vi "Main.vi"() -> ()   [LabVIEW 2019]
doc: "This template is for the Queued Message Handler design pattern.\n\nThe Event Handling Loop generates messages based on user interface actions.\n\nThe Message Handling Loop processes messages generated by the Event Handling Loop, or by other messages. The messages are string values, so new messages can be added easily to the Message Cases case structure in the Message Handling Loop. Each message cluster can also provide an optional value for Message Data, which is a variant that can be converted to whatever message-specific data is required."
uses:
  controls/UI Data.ctl
  support/Message Queue/Message Queue.lvlib
  <vilib>/Utility/error.llb/Error Cluster From Error Code.vi
  support/User Event - Stop/User Event - Stop.lvlib
  support/Message Queue/Enqueue Message (Single).vi
  <vilib>/ErrorRing/Error Ring.xnode
  <vilib>/Analysis/NI_AALBase.lvlib
  <vilib>/Instr/_visa.llb/VISA Configure Serial Port (Instr).vi
panel:
  in  "?":enum32{"PLSC-21/LDP-V", "BFS-VRM 03"}(tab)
  in  "Set Max. Duty Cycle":dbl
  out "Duty Cycle":dbl(slide) scale=0.0..0.15
  in  "Exit":bool
  in  "Start Laser":bool
  in  "Stop Laser":bool
  out "Display (Code)":string
  in  "Pulse Length (ns)":dbl(slide) scale=8.0..100.0
  in  "Set Pulse Length":bool
  in  "Voltage (mv)":dbl(slide) scale=0.0..10000.0
  in  "Set Precharger Voltage":bool
  in  "Rep. Rate (Hz)":dbl(slide) scale=0.0..1000.0
  in  "Modes":enum32{"Voltage Mode", "Current Mode"}(radio)
  in  "Current":u64(knob) scale=0.0..100.0
  out "Waveform":dbl[](graph)
  in  "Sample Rate":i32(slide) scale=0.0..8000.0
  out "LED":bool=TRUE
  in  "Save Settings\nPLCS":bool
  in  "Load Settings\nPLCS":bool
  in  "Save Settings BFS":bool
  in  "TEC Current Limit (A)":dbl(slide) scale=0.0..1.0
  in  "TEC KI":dbl(slide) scale=0.0..0.04
  in  "TEC KP":dbl(slide) scale=0.0..2.0
  in  "TEC Temperatur":dbl(knob) scale=0.0..70.0
  in  "VREF (V)":dbl(slide) scale=0.0..1.0
  in  "Load Settings BFS":bool
  out "Display (Code)":string
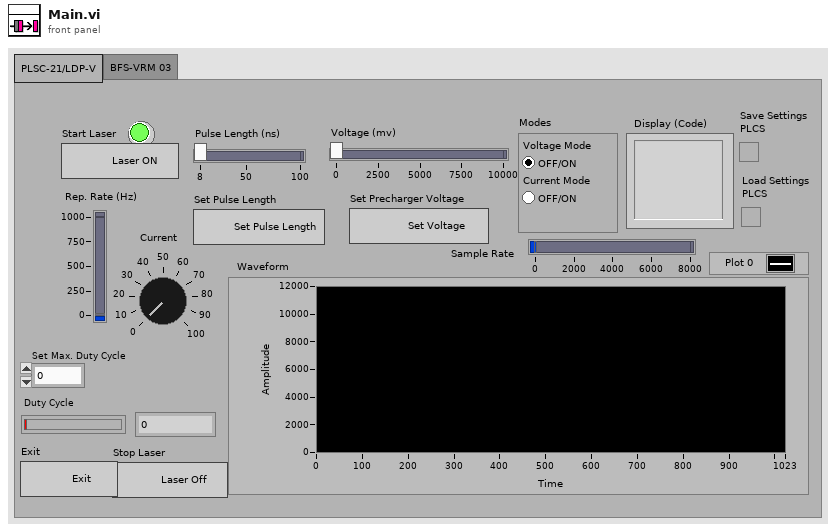
[diagram p1: front panel]
types:
  T1 = typedef "UI Data.ctl" = cluster{"Boolean <Replace Me>":bool, "String <Replace Me>":string, "Numeric <Replace Me>":dbl, "Do Something Ref":refnum<vi>, "Do Something Else Ref":refnum<vi>, "Data Display Ref":refnum<vi>, "Exit Button Ref":refnum<vi>}
  T2 = typedef "Message Queue.lvlib/All Message Queues.ctl" = cluster{"UI":refnum<queue>}
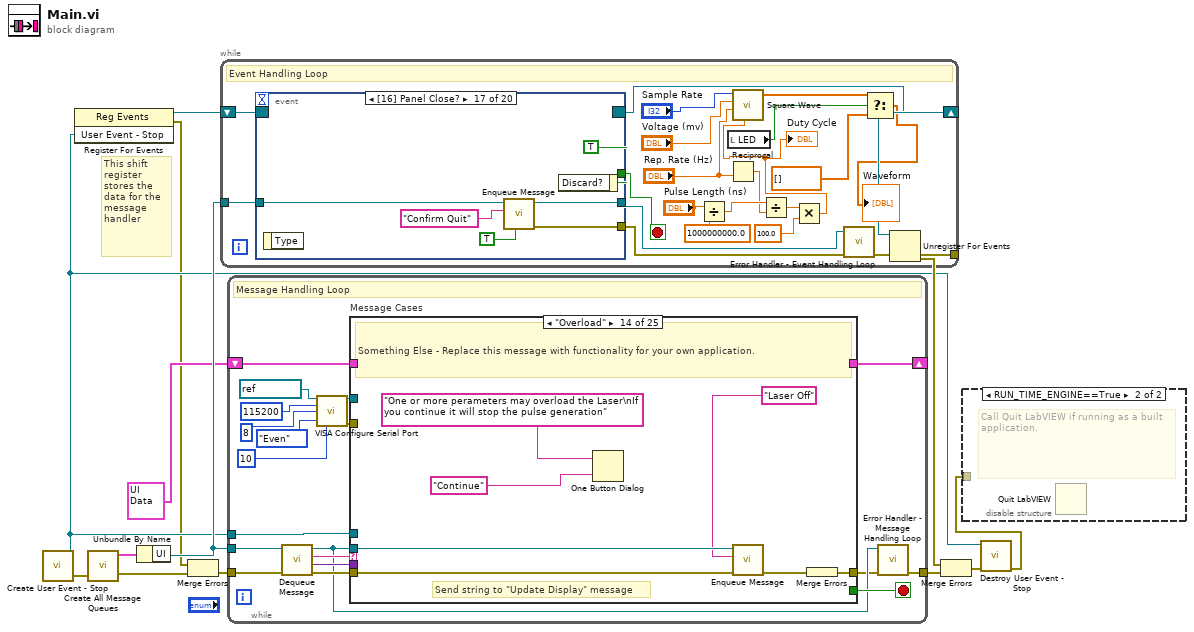
[diagram p0: block diagram]
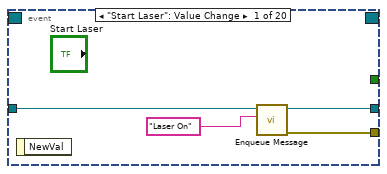
[diagram p3: hidden frame]
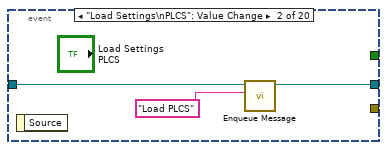
[diagram p4: hidden frame]
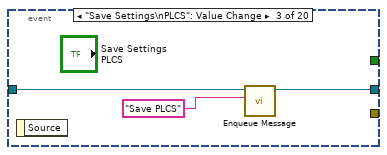
[diagram p5: hidden frame]
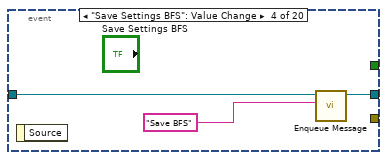
[diagram p6: hidden frame]
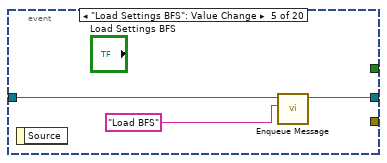
[diagram p7: hidden frame]
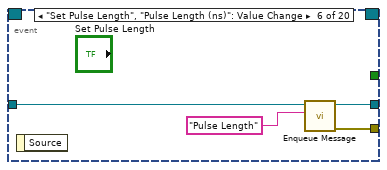
[diagram p8: hidden frame]
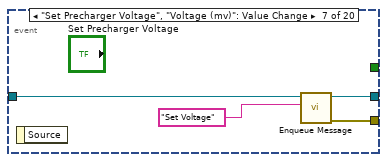
[diagram p9: hidden frame]
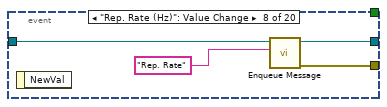
[diagram p10: hidden frame]
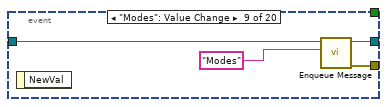
[diagram p11: hidden frame]
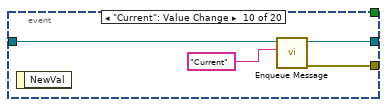
[diagram p12: hidden frame]
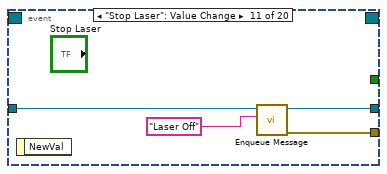
[diagram p13: hidden frame]
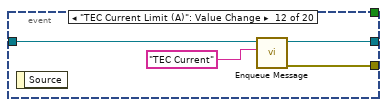
[diagram p14: hidden frame]
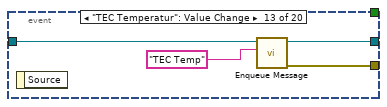
[diagram p15: hidden frame]
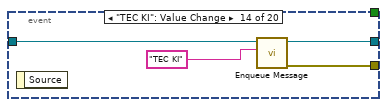
[diagram p16: hidden frame]
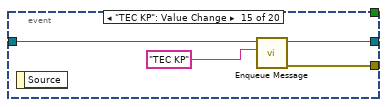
[diagram p17: hidden frame]
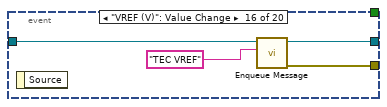
[diagram p18: hidden frame]
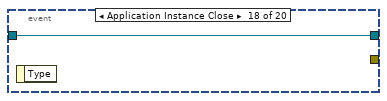
[diagram p19: hidden frame]
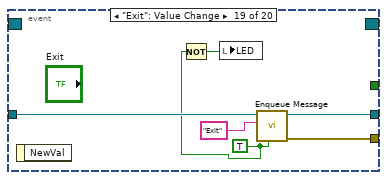
[diagram p20: hidden frame]
diagram:
  # "This shift register stores the data for the message handler"
  n1 = call "Create User Event - Stop.vi"() -> ("error out"=w11:errorcluster, "User Event - Stop"=w4:refnum<user-event>)  [unwired: 10 in]
  n2 = register-events(w4) -> (reference out=w5:refnum<event-registration>, error out=w2:errorcluster)  [unwired: 2 in]
  n3 = call "Create All Message Queues.vi"("error in (no error)"=w11) -> ("error out"=w15:errorcluster, "Message Queues out"=w14:T2)  [unwired: 9 in]
  n4 = Unbundle By Name(w14) -> ("UI"=w12:refnum<queue>)
  n5 = Merge Errors(w2, w15) -> (w3:errorcluster)
  n6 = while {
    tunnel: w12 -> [w36]
    shift-right: [w31] -> w8
    shift-left: w5 -> [w35]
    tunnel: [w33] -> w6
    stop <- w30 stop-if-true
    # "Event Handling Loop"
    n7 = event shown="[16] Panel Close?" {
      selector: w35 -> [_ _ _ _ _ _ _ _ _ _ _ _ _ _ _ _ _ _ _ _]
      dyn-events: [_ _ _ _ _ _ _ _ _ _ _ _ _ _ _ _ _ _ _ _] -> w31
      timeout: _ -> [_ _ _ _ _ _ _ _ _ _ _ _ _ _ _ _ _ _ _ _]
      tunnel: [_ _ _ _ _ _ _ _ _ _ _ _ _ _ _ _ _ _ _ TRUE ("Discard?")] -> w30
      tunnel: w36 -> [w40 w43 w46 w48 w51 w55 w60 w64 w68 w72 w76 w80 w84 w88 w92 w96 w101 w103 w109 w112]
      tunnel: [w37 _ _ _ _ w53 w58 w61 w65 w70 w73 w77 w81 w85 w89 w93 w100 _ w108 _] -> w34
      tunnel: [w39 w42 w45 w49 w52 w54 w59 w63 w67 w71 w75 w79 w83 w87 w91 w95 w99 w103 w107 w112] -> w32
      event "Start Laser": Value Change {
        n8 = event-data() -> ()  [unwired: 1 in, 1 out]
        n9 = call-poly "Enqueue Message.vi"("Message"="Laser On", "Message Queue"=w40) -> ("error out"=w37:errorcluster, "dup Message Queue"=w39:refnum<queue>)  [unwired: 8 in]
      }
      event "Load Settings\nPLCS": Value Change {
        n10 = event-data() -> ()  [unwired: 1 in, 1 out]
        n11 = call-poly "Enqueue Message.vi"("Message"="Load PLCS", "Message Queue"=w43) -> ("dup Message Queue"=w42:refnum<queue>)  [unwired: 8 in, 1 out]
      }
      event "Save Settings\nPLCS": Value Change {
        n12 = event-data() -> ()  [unwired: 1 in, 1 out]
        n13 = call-poly "Enqueue Message.vi"("Message"="Save PLCS", "Message Queue"=w46) -> ("dup Message Queue"=w45:refnum<queue>)  [unwired: 8 in, 1 out]
      }
      event "Save Settings BFS": Value Change {
        n14 = event-data() -> ()  [unwired: 1 in, 1 out]
        n15 = call-poly "Enqueue Message.vi"("Message"="Save BFS", "Message Queue"=w48) -> ("dup Message Queue"=w49:refnum<queue>)  [unwired: 8 in, 1 out]
      }
      event "Load Settings BFS": Value Change {
        n16 = event-data() -> ()  [unwired: 1 in, 1 out]
        n17 = call-poly "Enqueue Message.vi"("Message"="Load BFS", "Message Queue"=w51) -> ("dup Message Queue"=w52:refnum<queue>)  [unwired: 8 in, 1 out]
      }
      event "Set Pulse Length", "Pulse Length (ns)": Value Change {
        n18 = event-data() -> ()  [unwired: 1 in, 1 out]
        n19 = call-poly "Enqueue Message.vi"("Message"="Pulse Length", "Message Queue"=w55) -> ("error out"=w53:errorcluster, "dup Message Queue"=w54:refnum<queue>)  [unwired: 8 in]
      }
      event "Set Precharger Voltage", "Voltage (mv)": Value Change {
        n20 = event-data() -> ()  [unwired: 1 in, 1 out]
        n21 = call-poly "Enqueue Message.vi"("Message"="Set Voltage", "Message Queue"=w60) -> ("error out"=w58:errorcluster, "dup Message Queue"=w59:refnum<queue>)  [unwired: 8 in]
      }
      event "Rep. Rate (Hz)": Value Change {
        n22 = event-data() -> ()  [unwired: 1 in, 1 out]
        n23 = call-poly "Enqueue Message.vi"("Message"="Rep. Rate", "Message Queue"=w64) -> ("error out"=w61:errorcluster, "dup Message Queue"=w63:refnum<queue>)  [unwired: 8 in]
      }
      event "Modes": Value Change {
        n24 = event-data() -> ()  [unwired: 1 in, 1 out]
        n25 = call-poly "Enqueue Message.vi"("Message"="Modes", "Message Queue"=w68) -> ("error out"=w65:errorcluster, "dup Message Queue"=w67:refnum<queue>)  [unwired: 8 in]
      }
      event "Current": Value Change {
        n26 = event-data() -> ()  [unwired: 1 in, 1 out]
        n27 = call-poly "Enqueue Message.vi"("Message"="Current", "Message Queue"=w72) -> ("error out"=w70:errorcluster, "dup Message Queue"=w71:refnum<queue>)  [unwired: 8 in]
      }
      event "Stop Laser": Value Change {
        n28 = event-data() -> ()  [unwired: 1 in, 1 out]
        n29 = call-poly "Enqueue Message.vi"("Message"="Laser Off", "Message Queue"=w76) -> ("error out"=w73:errorcluster, "dup Message Queue"=w75:refnum<queue>)  [unwired: 8 in]
      }
      event "TEC Current Limit (A)": Value Change {
        n30 = event-data() -> ()  [unwired: 1 in, 1 out]
        n31 = call-poly "Enqueue Message.vi"("Message"="TEC Current", "Message Queue"=w80) -> ("error out"=w77:errorcluster, "dup Message Queue"=w79:refnum<queue>)  [unwired: 8 in]
      }
      event "TEC Temperatur": Value Change {
        n32 = event-data() -> ()  [unwired: 1 in, 1 out]
        n33 = call-poly "Enqueue Message.vi"("Message"="TEC Temp", "Message Queue"=w84) -> ("error out"=w81:errorcluster, "dup Message Queue"=w83:refnum<queue>)  [unwired: 8 in]
      }
      event "TEC KI": Value Change {
        n34 = event-data() -> ()  [unwired: 1 in, 1 out]
        n35 = call-poly "Enqueue Message.vi"("Message"="TEC KI", "Message Queue"=w88) -> ("error out"=w85:errorcluster, "dup Message Queue"=w87:refnum<queue>)  [unwired: 8 in]
      }
      event "TEC KP": Value Change {
        n36 = event-data() -> ()  [unwired: 1 in, 1 out]
        n37 = call-poly "Enqueue Message.vi"("Message"="TEC KP", "Message Queue"=w92) -> ("error out"=w89:errorcluster, "dup Message Queue"=w91:refnum<queue>)  [unwired: 8 in]
      }
      event "VREF (V)": Value Change {
        n38 = event-data() -> ()  [unwired: 1 in, 1 out]
        n39 = call-poly "Enqueue Message.vi"("Message"="TEC VREF", "Message Queue"=w96) -> ("error out"=w93:errorcluster, "dup Message Queue"=w95:refnum<queue>)  [unwired: 8 in]
      }
      event Panel Close? {
        n40 = event-data() -> ()  [unwired: 1 in, 1 out]
        n41 = call-poly "Enqueue Message.vi"("Priority Message? (F)"=TRUE, "Message"="Confirm Quit", "Message Queue"=w101) -> ("error out"=w100:errorcluster, "dup Message Queue"=w99:refnum<queue>)  [unwired: 7 in]
        n42 = event-data("Discard?"=TRUE) -> ()  [unwired: 1 in, 1 out]
      }
      event Application Instance Close {
        n43 = event-data() -> ()  [unwired: 1 in, 1 out]
      }
      event "Exit": Value Change {
        w104 = TRUE ("Priority Message? (F)")
        n44 = event-data() -> ()  [unwired: 1 in, 1 out]
        n45 = Not(x=w104) -> (.not. x?=w105:bool)
        n46 = local write "LED"(w105) -> ()
        n47 = call-poly "Enqueue Message.vi"("Priority Message? (F)"=w104, "Message"="Exit", "Message Queue"=w109) -> ("error out"=w108:errorcluster, "dup Message Queue"=w107:refnum<queue>)  [unwired: 7 in]
      }
      event User Event {
        n48 = event-data() -> ()  [unwired: 1 in, 1 out]
        n49 = local write "Display (Code)"("\"Exit\" button pressed/COM Released" ("VI Stopped")) -> ()
      }
    }
    n50 = Divide(x="Pulse Length (ns)", y=1000000000.0) -> (x/y=w26:dbl)
    n51 = local read "LED"() -> (w19:bool)
    n52 = Reciprocal(x="Rep. Rate (Hz)") -> (1/x=w25:dbl)
    n53 = Divide(x=w26, y=w25) -> (x/y=w24:dbl)
    n54 = Multiply(x=w24, y=100.0) -> (x*y=w17:dbl)
    "Duty Cycle" <- w17
    n55 = call <vilib>:"Square Wave.vi"("samples"="Sample Rate", "amplitude"="Voltage (mv)", "frequency"="Rep. Rate (Hz)", "duty cycle (%)"=w17) -> ("square wave"=w20:dbl[])  [unwired: 2 in, 2 out]
    n56 = call "Error Handler - Event Handling Loop.vi"("error in (no error)"=w34, "Message Queue"=w32) -> ("dup error in"=w33:errorcluster)  [unwired: 8 in, 1 out]
    n57 = Select(t=w20, s=w19, f=dbl[] [] ("History Data")) -> (s? t:f=→"Waveform":dbl[])
  }
  n58 = while {
    tunnel: w12 -> [w123]
    shift-right: [w130] -> _
    shift-left: T1 {"Boolean <Replace Me>"=FALSE, "String <Replace Me>"="", "Numeric <Replace Me>"=0.0, "Do Something Ref"=refnum, "Do Something Else Ref"=refnum, "Data Display Ref"=refnum, "Exit Button Ref"=refnum} ("Data Cluster") -> [w131]
    tunnel: w4 -> [w128]
    tunnel: w3 -> [w127]
    tunnel: [w121] -> w13
    stop <- w129 stop-if-true
    # "Message Handling Loop"
    n59 = call "Dequeue Message.vi"("error in (no error)"=w127, "Message Queue"=w123) -> ("error out"=w126:errorcluster, "Message Data"=w124:variant, "Message"=w125:string, "dup Message Queue"=w122:refnum<queue>)  [unwired: 6 in]
    n60 = call-poly "VISA Configure Serial Port"("VISA resource name"=refnum<visa-resource-name> "COM4", "baud rate (9600)"=u32 115200, "data bits (8)"=u16 8, "parity (0:none)"=enum16{"None", "Odd", "Even", "Mark", "Space"}."Even", "stop bits (10: 1 bit)"=u16 10) -> ("VISA resource name out"=w114:refnum<visa-resource-name>, "error out"=w113:errorcluster)  [unwired: 9 in]
    n61 = case "Message Cases" shown="\"Overload\"" w125 {
      selector: w125 -> [_ _ _ _ _ _ _ _ _ _ _ _ _ _ _ _ _ _ _ _ _ _ _ _ w434]
      tunnel: w122 -> [w136 w160 w175 w195 w214 w220 w245 w263 w281 w299 w317 w330 w344 w352 _ _ _ _ _ _ _ w412 _ w433 _]
      tunnel: w126 -> [w144 w161 w177 w197 w216 w222 w247 w265 w283 w301 w319 w332 w346 w354 w364 w372 w380 w388 w393 w400 w409 w416 w419 w426 _]
      tunnel: [w145 w163 w176 w196 w215 w221 w246 w264 w282 w300 w318 w333 w347 w355 w364 w372 w380 w388 w394 w401 w403 w414 w417 w429 w435] -> w120
      tunnel: w131 -> [w143 w147 w180 w185 w219 w231 w249 w267 w285 w303 w321 w334 w348 w356 w363 w371 w379 w387 w395 w402 w408 w415 w418 w432 w436]
      tunnel: [w142 w147 w180 w185 w219 w231 w249 w267 w285 w303 w321 w334 w348 w356 w363 w371 w379 w387 w395 w402 w408 w415 w418 w432 w436] -> w130
      tunnel: [_ _ _ _ _ _ _ _ _ _ _ _ _ _ _ _ _ _ _ _ _ _ _ TRUE _] -> w129
      tunnel: w124 -> [_ _ _ _ _ _ _ _ _ _ _ _ _ _ _ _ _ _ w392 w399 w407 _ _ w423 _]
      tunnel: w128 -> [_ _ _ _ _ _ _ _ _ _ _ _ _ _ _ _ _ _ _ _ _ _ _ w428 _]
      tunnel: w114 -> [_ w168 w179 w203 w213 w230 _ _ _ _ _ w328 w340 _ _ _ _ _ _ _ _ _ _ w422 _]
      tunnel: w113 -> [_ w167 w178 w202 w212 w229 _ _ _ _ _ w327 w339 _ _ _ _ _ _ _ _ _ _ w421 _]
      frame "Initialize" {
        w132 = "Initial Message" ("Initial Message")
        # "Bundle control references and a sample string value."
        # "Initialize - All initialization work should take place in this message, since other loops can potentially enqueue messages that execute immediately after this one."
        n62 = control-ref of="Start Laser"() -> (w141:refnum<vi>)
        n63 = control-ref of="Stop Laser"() -> (w140:refnum<vi>)
        n64 = control-ref of="Exit"() -> (w138:refnum<vi>)
        n65 = control-ref of="Display (Code)"() -> (w139:refnum<vi>)
        n66 = String Length(string=w132) -> (length=w134:i32)
        n67 = Less Than 0?(x=w134) -> (x < 0?=w133:bool)
        n68 = Bundle By Name(cluster=w143, "Do Something Ref"=w141, "Do Something Else Ref"=w140, "Data Display Ref"=w139, "Exit Button Ref"=w138, "String <Replace Me>"=w132) -> (w142:T1)
        n69 = local write "LED"(w133) -> ()
        n70 = property on="Waveform" class="WFChart (strict)"("History Data"=dbl[] []) -> ()  [unwired: 2 in, 2 out]
        n71 = call-poly "Enqueue Message.vi"("error in (no error)"=w144, "Message Data"=w132, "Message"="Update Display", "Message Queue"=w136) -> ("error out"=w145:errorcluster)  [unwired: 6 in, 1 out]
      }
      frame "Pulse Length" {
        n72 = local read "Pulse Length (ns)"() -> (w162:dbl)
        n73 = local read "Duty Cycle"() -> (w154:dbl)
        n74 = Concatenate Strings("Laseroff" ("Message"), "\r") -> (w148:string)
        n75 = Number To Decimal String(number=w162) -> (decimal integer string=w165:string)  [unwired: 1 in]
        n76 = Greater Or Equal?(x=w154, y="Set Max. Duty Cycle") -> (x >= y?=w155:bool)
        n77 = In Range and Coerce(upper limit="Set Max. Duty Cycle", x=w154, lower limit=0.0) -> (In Range?=w158:bool)  [unwired: 1 out]
        n78 = Select(t="Overload" ("Message"), s=w155, f="Update Display" ("Message")) -> (s? t:f=w153:string)
        n79 = Concatenate Strings("spulse ", w165, "\r") -> (w157:string)
        n80 = Select(t=w157, s=w158, f=w148) -> (s? t:f=w156:string)
        n81 = VISA Write(VISA resource name=w168, write buffer=w156, error in (no error)=w167) -> ()  [unwired: 3 out]
        n82 = call-poly "Enqueue Message.vi"("error in (no error)"=w161, "Message Data"=w156, "Message"=w153, "Message Queue"=w160) -> ("error out"=w163:errorcluster)  [unwired: 6 in, 1 out]
      }
      frame "Set Voltage" {
        n83 = local read "Voltage (mv)"() -> (w169:dbl)
        n84 = Number To Decimal String(number=w169) -> (decimal integer string=w172:string)  [unwired: 1 in]
        n85 = Concatenate Strings("svoltage  ", w172, "\r") -> (w170:string)
        n86 = VISA Write(VISA resource name=w179, write buffer=w170, error in (no error)=w178) -> ()  [unwired: 3 out]
        n87 = call-poly "Enqueue Message.vi"("error in (no error)"=w177, "Message Data"=w170, "Message"="Update Display", "Message Queue"=w175) -> ("error out"=w176:errorcluster)  [unwired: 6 in, 1 out]
      }
      frame "Rep. Rate" {
        n88 = local read "Set Max. Duty Cycle"() -> (w181:dbl)
        n89 = local read "Rep. Rate (Hz)"() -> (w198:dbl)
        n90 = local read "Duty Cycle"() -> (w186:dbl)
        n91 = In Range and Coerce(upper limit=w181, x=w186, lower limit=0.0) -> (In Range?=w193:bool)  [unwired: 1 out]
        n92 = Concatenate Strings("laseroff ", "\r") -> (w189:string)
        n93 = Number To Decimal String(number=w198) -> (decimal integer string=w200:string)  [unwired: 1 in]
        n94 = Greater Or Equal?(x=w186, y=w181) -> (x >= y?=w187:bool)
        n95 = Select(t="Overload" ("Message"), s=w187, f="Update Display" ("Message")) -> (s? t:f=w183:string)
        n96 = Concatenate Strings("sreprate  ", w200, "\r") -> (w192:string)
        n97 = Select(t=w192, s=w193, f=w189) -> (s? t:f=w188:string)
        n98 = VISA Write(VISA resource name=w203, write buffer=w188, error in (no error)=w202) -> ()  [unwired: 3 out]
        n99 = call-poly "Enqueue Message.vi"("error in (no error)"=w197, "Message Data"=w188, "Message"=w183, "Message Queue"=w195) -> ("error out"=w196:errorcluster)  [unwired: 6 in, 1 out]
      }
      frame "Modes" {
        n100 = Equal To 0?(x="Modes") -> (x = 0?=w218:bool)
        n101 = Select(t=1, s=w218, f=2) -> (s? t:f=w209:i32)
        n102 = Number To Decimal String(number=w209) -> (decimal integer string=w208:string)  [unwired: 1 in]
        n103 = Concatenate Strings("smode ", w208, "\r") -> (w204:string)
        n104 = VISA Write(VISA resource name=w213, write buffer=w204, error in (no error)=w212) -> ()  [unwired: 3 out]
        n105 = call-poly "Enqueue Message.vi"("error in (no error)"=w216, "Message Data"=w204, "Message"="Update Display", "Message Queue"=w214) -> ("error out"=w215:errorcluster)  [unwired: 6 in, 1 out]
      }
      frame "Current" {
        n106 = Number To Decimal String(number="Current") -> (decimal integer string=w228:string)  [unwired: 1 in]
        n107 = Concatenate Strings("scurrent  ", w228, "\r") -> (w224:string)
        n108 = VISA Write(VISA resource name=w230, write buffer=w224, error in (no error)=w229) -> ()  [unwired: 3 out]
        n109 = call-poly "Enqueue Message.vi"("error in (no error)"=w222, "Message Data"=w224, "Message"="Update Display", "Message Queue"=w220) -> ("error out"=w221:errorcluster)  [unwired: 6 in, 1 out]
      }
      frame "TEC Current" {
        n110 = local read "TEC Current Limit (A)"() -> (w244:dbl)
        n111 = call-poly "VISA Configure Serial Port"("VISA resource name"=refnum<visa-resource-name> "COM3", "baud rate (9600)"=u32 115200, "data bits (8)"=u16 8, "parity (0:none)"=enum16{"None", "Odd", "Even", "Mark", "Space"}."Even", "stop bits (10: 1 bit)"=u16 10) -> ("VISA resource name out"=w233:refnum<visa-resource-name>, "error out"=w232:errorcluster)  [unwired: 9 in]
        n112 = Number To Fractional String(number=w244, precision (6)=2) -> (F-format string=w243:string)  [unwired: 2 in]
        n113 = Concatenate Strings("simax  ", w243, "\r") -> (w239:string)
        n114 = VISA Write(VISA resource name=w233, write buffer=w239, error in (no error)=w232) -> ()  [unwired: 3 out]
        n115 = call-poly "Enqueue Message.vi"("error in (no error)"=w247, "Message Data"=w239, "Message"="Display 2", "Message Queue"=w245) -> ("error out"=w246:errorcluster)  [unwired: 6 in, 1 out]
      }
      frame "TEC Temp" {
        w259 = "stsoll  "  # stsoll
        n116 = local read "TEC Temperatur"() -> (w262:dbl)
        n117 = call-poly "VISA Configure Serial Port"("VISA resource name"=refnum<visa-resource-name> "COM3", "baud rate (9600)"=u32 115200, "data bits (8)"=u16 8, "parity (0:none)"=enum16{"None", "Odd", "Even", "Mark", "Space"}."Even", "stop bits (10: 1 bit)"=u16 10) -> ("VISA resource name out"=w251:refnum<visa-resource-name>, "error out"=w250:errorcluster)  [unwired: 9 in]
        n118 = Number To Fractional String(number=w262, precision (6)=0) -> (F-format string=w261:string)  [unwired: 2 in]
        n119 = Concatenate Strings(w259, w261, "\r") -> (w257:string)
        n120 = VISA Write(VISA resource name=w251, write buffer=w257, error in (no error)=w250) -> ()  [unwired: 3 out]
        n121 = call-poly "Enqueue Message.vi"("error in (no error)"=w265, "Message Data"=w257, "Message"="Display 2", "Message Queue"=w263) -> ("error out"=w264:errorcluster)  [unwired: 6 in, 1 out]
      }
      frame "TEC KI" {
        w277 = "ski  "  # ski
        n122 = local read "TEC KI"() -> (w280:dbl)
        n123 = call-poly "VISA Configure Serial Port"("VISA resource name"=refnum<visa-resource-name> "COM3", "baud rate (9600)"=u32 115200, "data bits (8)"=u16 8, "parity (0:none)"=enum16{"None", "Odd", "Even", "Mark", "Space"}."Even", "stop bits (10: 1 bit)"=u16 10) -> ("VISA resource name out"=w269:refnum<visa-resource-name>, "error out"=w268:errorcluster)  [unwired: 9 in]
        n124 = Number To Fractional String(number=w280, precision (6)=2) -> (F-format string=w279:string)  [unwired: 2 in]
        n125 = Concatenate Strings(w277, w279, "\r") -> (w275:string)
        n126 = VISA Write(VISA resource name=w269, write buffer=w275, error in (no error)=w268) -> ()  [unwired: 3 out]
        n127 = call-poly "Enqueue Message.vi"("error in (no error)"=w283, "Message Data"=w275, "Message"="Display 2", "Message Queue"=w281) -> ("error out"=w282:errorcluster)  [unwired: 6 in, 1 out]
      }
      frame "TEC KP" {
        w295 = "skp  "  # skp
        n128 = local read "TEC KP"() -> (w298:dbl)
        n129 = call-poly "VISA Configure Serial Port"("VISA resource name"=refnum<visa-resource-name> "COM3", "baud rate (9600)"=u32 115200, "data bits (8)"=u16 8, "parity (0:none)"=enum16{"None", "Odd", "Even", "Mark", "Space"}."Even", "stop bits (10: 1 bit)"=u16 10) -> ("VISA resource name out"=w287:refnum<visa-resource-name>, "error out"=w286:errorcluster)  [unwired: 9 in]
        n130 = Number To Fractional String(number=w298, precision (6)=2) -> (F-format string=w297:string)  [unwired: 2 in]
        n131 = Concatenate Strings(w295, w297, "\r") -> (w293:string)
        n132 = VISA Write(VISA resource name=w287, write buffer=w293, error in (no error)=w286) -> ()  [unwired: 3 out]
        n133 = call-poly "Enqueue Message.vi"("error in (no error)"=w301, "Message Data"=w293, "Message"="Display 2", "Message Queue"=w299) -> ("error out"=w300:errorcluster)  [unwired: 6 in, 1 out]
      }
      frame "TEC VREF" {
        w313 = "svref "  # svref
        n134 = local read "VREF (V)"() -> (w316:dbl)
        n135 = call-poly "VISA Configure Serial Port"("VISA resource name"=refnum<visa-resource-name> "COM3", "baud rate (9600)"=u32 115200, "data bits (8)"=u16 8, "parity (0:none)"=enum16{"None", "Odd", "Even", "Mark", "Space"}."Even", "stop bits (10: 1 bit)"=u16 10) -> ("VISA resource name out"=w305:refnum<visa-resource-name>, "error out"=w304:errorcluster)  [unwired: 9 in]
        n136 = Number To Fractional String(number=w316, precision (6)=2) -> (F-format string=w315:string)  [unwired: 2 in]
        n137 = Concatenate Strings(w313, w315, "\r") -> (w311:string)
        n138 = VISA Write(VISA resource name=w305, write buffer=w311, error in (no error)=w304) -> ()  [unwired: 3 out]
        n139 = call-poly "Enqueue Message.vi"("error in (no error)"=w319, "Message Data"=w311, "Message"="Display 2", "Message Queue"=w317) -> ("error out"=w318:errorcluster)  [unwired: 6 in, 1 out]
      }
      frame "Laser On" {
        # "Send string to \"Update Display\" message"
        # "Something - Replace this message with functionality for your own application."
        n140 = Concatenate Strings("laseron", "\r") -> (w323:string)
        n141 = String Length(string=w323) -> (length=w322:i32)
        n142 = VISA Write(VISA resource name=w328, write buffer=w323, error in (no error)=w327) -> ()  [unwired: 3 out]
        n143 = Greater Than 0?(x=w322) -> (x > 0?=→"LED":bool)
        n144 = call-poly "Enqueue Message.vi"("error in (no error)"=w332, "Message Data"=w323, "Message"="Update Display", "Message Queue"=w330) -> ("error out"=w331:errorcluster)  [unwired: 6 in, 1 out]
        n145 = Merge Errors(w331) -> (w333:errorcluster)
      }
      frame "Laser Off" {
        # "Send string to \"Update Display\" message"
        # "Something Else - Replace this message with functionality for your own application."
        n146 = Concatenate Strings("laseroff", "\r") -> (w335:string)
        n147 = VISA Write(VISA resource name=w340, write buffer=w335, error in (no error)=w339) -> ()  [unwired: 3 out]
        n148 = String Length(string=w335) -> (length=w337:i32)
        n149 = Less Than 0?(x=w337) -> (x < 0?=w336:bool)
        n150 = local write "LED"(w336) -> ()
        n151 = call-poly "Enqueue Message.vi"("error in (no error)"=w346, "Message Data"=w335, "Message"="Update Display", "Message Queue"=w344) -> ("error out"=w345:errorcluster)  [unwired: 6 in, 1 out]
        n152 = property on="Waveform" class="WFChart (strict)"("History Data"=dbl[] []) -> ()  [unwired: 2 in, 2 out]
        n153 = Merge Errors(w345) -> (w347:errorcluster)
      }
      frame "Overload" {
        # "Send string to \"Update Display\" message"
        # "Something Else - Replace this message with functionality for your own application."
        n154 = One Button Dialog(message="One or more perameters may overload the Laser\nIf you continue it will stop the pulse generation" ("Message"), button name ("OK")="Continue" ("Message")) -> ()  [unwired: 1 out]
        n155 = call-poly "Enqueue Message.vi"("error in (no error)"=w354, "Message"="Laser Off", "Message Queue"=w352) -> ("error out"=w353:errorcluster)  [unwired: 7 in, 1 out]
        n156 = Merge Errors(w353) -> (w355:errorcluster)
      }
      frame "Save BFS" {
        n157 = Merge Signals("TEC Temperatur", "VREF (V)", "TEC KI", "TEC KP", "TEC Current Limit (A)") -> (w362:dynamicdata)
        n158 = call "Write To Measurement File"("Signals"=w362) -> ()  [unwired: 16 in, 3 out]
      }
      frame "Save PLCS" {
        n159 = local read "Pulse Length (ns)"() -> (w366:dbl)
        n160 = local read "Rep. Rate (Hz)"() -> (w369:dbl)
        n161 = local read "Voltage (mv)"() -> (w367:dbl)
        n162 = local read "Set Max. Duty Cycle"() -> (w365:dbl)
        n163 = local read "Current"() -> (w368:u64)
        n164 = Merge Signals(w369, w367, w366, w368, w365) -> (w370:dynamicdata)
        n165 = call "Write To Measurement File2"("Signals"=w370) -> ()  [unwired: 16 in, 3 out]
      }
      frame "Load BFS" {
        n166 = call "Read From Measurement File"() -> ("Signals"=w373:dynamicdata)  [unwired: 6 in, 5 out]
        n167 = Split Signals(w373) -> (w374:dynamicdata, w375:dynamicdata, w378:dynamicdata, w376:dynamicdata, w377:dynamicdata)  [unwired: 5 in]
        n168 = property on="TEC Current Limit (A)" class="Slide (strict)"("Value"=w374) -> ()  [unwired: 2 in, 2 out]
        n169 = property on="TEC KP" class="Slide (strict)"("Value"=w375) -> ()  [unwired: 2 in, 2 out]
        n170 = property on="TEC KI" class="Slide (strict)"("Value"=w378) -> ()  [unwired: 2 in, 2 out]
        n171 = property on="VREF (V)" class="Slide (strict)"("Value"=w376) -> ()  [unwired: 2 in, 2 out]
        n172 = property on="TEC Temperatur" class="Knob (strict)"("Value"=w377) -> ()  [unwired: 2 in, 2 out]
      }
      frame "Load PLCS" {
        n173 = call "Read From Measurement File2"() -> ("Signals"=w386:dynamicdata)  [unwired: 6 in, 5 out]
        n174 = Split Signals(w386) -> (w385:dynamicdata, w384:dynamicdata, w383:dynamicdata, w382:dynamicdata, w381:dynamicdata)  [unwired: 5 in]
        n175 = property on="Rep. Rate (Hz)" class="Slide (strict)"("Value"=w385) -> ()  [unwired: 2 in, 2 out]
        n176 = property on="Current" class="Knob (strict)"("Value"=w382) -> ()  [unwired: 2 in, 2 out]
        n177 = property on="Pulse Length (ns)" class="Slide (strict)"("Value"=w384) -> ()  [unwired: 2 in, 2 out]
        n178 = property on="Voltage (mv)" class="Slide (strict)"("Value"=w383) -> ()  [unwired: 2 in, 2 out]
        n179 = property on="Set Max. Duty Cycle" class="DigNum (strict)"("Value"=w381) -> ()  [unwired: 2 in, 2 out]
      }
      frame "Update Display" {
        # "#CodeRecommended - If you wish to decouple the Message Handling Loop from your user interface, consider creating User Events (like the \"Stop\" event in this VI) to message the Event Handling Loop whenever the user interface needs updating."
        # "Update Display - Convert the message data to a string to display in the Data Display indicator."
        n180 = Variant To Data(error in=w393, type="", Variant=w392) -> (data=→"Display (Code)":string, error out=w390:errorcluster)
        n181 = Merge Errors(w390) -> (w394:errorcluster)
      }
      frame "Display 2" {
        # "#CodeRecommended - If you wish to decouple the Message Handling Loop from your user interface, consider creating User Events (like the \"Stop\" event in this VI) to message the Event Handling Loop whenever the user interface needs updating."
        # "Update Display - Convert the message data to a string to display in the Data Display indicator."
        n182 = Variant To Data(error in=w400, type="", Variant=w399) -> (data=→"Display (Code)":string, error out=w397:errorcluster)
        n183 = Merge Errors(w397) -> (w401:errorcluster)
      }
      frame "Error" {
        # "#CodeRecommended - If you ever change the name of this \"Error\" message, you'll need to update the name in the Check Loop Error.vi as well."
        # "#CodeRecommended - Consider creating a system for logging errors in some way. These errors are for notification purposes only. Handling of specific errors should be performed in the message frames that generated the error."
        # "Error - Display an error dialog. This message is sent by the \"Error Handler\" VIs at the end of other loops in this application."
        n184 = Variant To Data(error in=w409, type=errorcluster {"status"=FALSE, "code"=0, "source"=""} ("error constant"), Variant=w407) -> (data=w405:errorcluster, error out=w404:errorcluster)
        n185 = call <vilib>:"Simple Error Handler.vi"("error in (no error)"=w405) -> ()  [unwired: 4 in, 5 out]
        n186 = Merge Errors(w404) -> (w403:errorcluster)
      }
      frame "Confirm Quit" {
        # "#CodeNeeded - If you want to provide an \"Are you sure\" dialog (or some other notification) before the application exits, place that code here. This message is typically sent from a Panel Close? event."
        # "Confirm Quit - Message that can confirm whether or not the user wants to exit the application."
        n187 = call-poly "Enqueue Message.vi"("Priority Message? (F)"=TRUE, "error in (no error)"=w416, "Message"="Exit", "Message Queue"=w412) -> ("error out"=w413:errorcluster)  [unwired: 6 in, 1 out]
        n188 = Merge Errors(w413) -> (w414:errorcluster)
      }
      frame "---Copy This Frame---" {
        # "Duplicate this frame when creating new messages.  Change this comment in the duplicated frame to describe this message."
        n189 = Merge Errors(w419) -> (w417:errorcluster)
      }
      frame "Exit" {
        # "Stop the VI"
        # "Release the message queue reference"
        # "Exit - Exit the application."
        n190 = Variant To Data(type=errorcluster {"status"=FALSE, "code"=0, "source"=""} ("error constant"), Variant=w423) -> (data=w424:errorcluster)  [unwired: 1 in, 1 out]
        n191 = VISA Close(VISA resource name=w422, error in (no error)=w421) -> ()  [unwired: 1 out]
        n192 = call <vilib>:"Simple Error Handler.vi"("error in (no error)"=w424) -> ()  [unwired: 4 in, 5 out]
        n193 = call "Fire User Event - Stop.vi"("User Event - Stop"=w428) -> ("error out"=w427:errorcluster)  [unwired: 10 in]
        n194 = Release Queue(queue=w433, error in (no error)=w426) -> (error out=w430:errorcluster)  [unwired: 1 in, 2 out]
        n195 = property on="Waveform" class="WFChart (strict)"("History Data"=dbl[] []) -> ()  [unwired: 2 in, 2 out]
        n196 = Merge Errors(w427, w430) -> (w429:errorcluster)
      }
      frame Default {
        # "'Default' case only runs if there is a message that isn't defined in any of the other cases.  Output a programming error."
        n197 = xnode "Error Ring"("parameter 0"=w434) -> ("error out"=w435:errorcluster)
      }
    }
    n198 = call "Error Handler - Message Handling Loop.vi"("error in (no error)"=w120, "Message Queue"=w122) -> ("dup error in"=w121:errorcluster)  [unwired: 8 in, 1 out]
  }
  n199 = Unregister For Events(event registration refnum=w8, error in=w6) -> (error out=w9:errorcluster)
  n200 = Merge Errors(w9, w13) -> (w10:errorcluster)
  n201 = call "Destroy User Event - Stop.vi"("error in (no error)"=w10, "User Event - Stop"=w4) -> ("error out"=w1:errorcluster)  [unwired: 9 in]
  n202 = disable-structure shown="RUN_TIME_ENGINE==True" {
    disable-tunnel: w1 -> [_ _]
    frame condition #0 (active) {
    }
    frame condition #1 {
      # "Call Quit LabVIEW if running as a built application."
      n203 = Quit LabVIEW() -> ()  [unwired: 1 in]
    }
  }
